vi "Rectifier Log Process.vi"   [LabVIEW 2019]
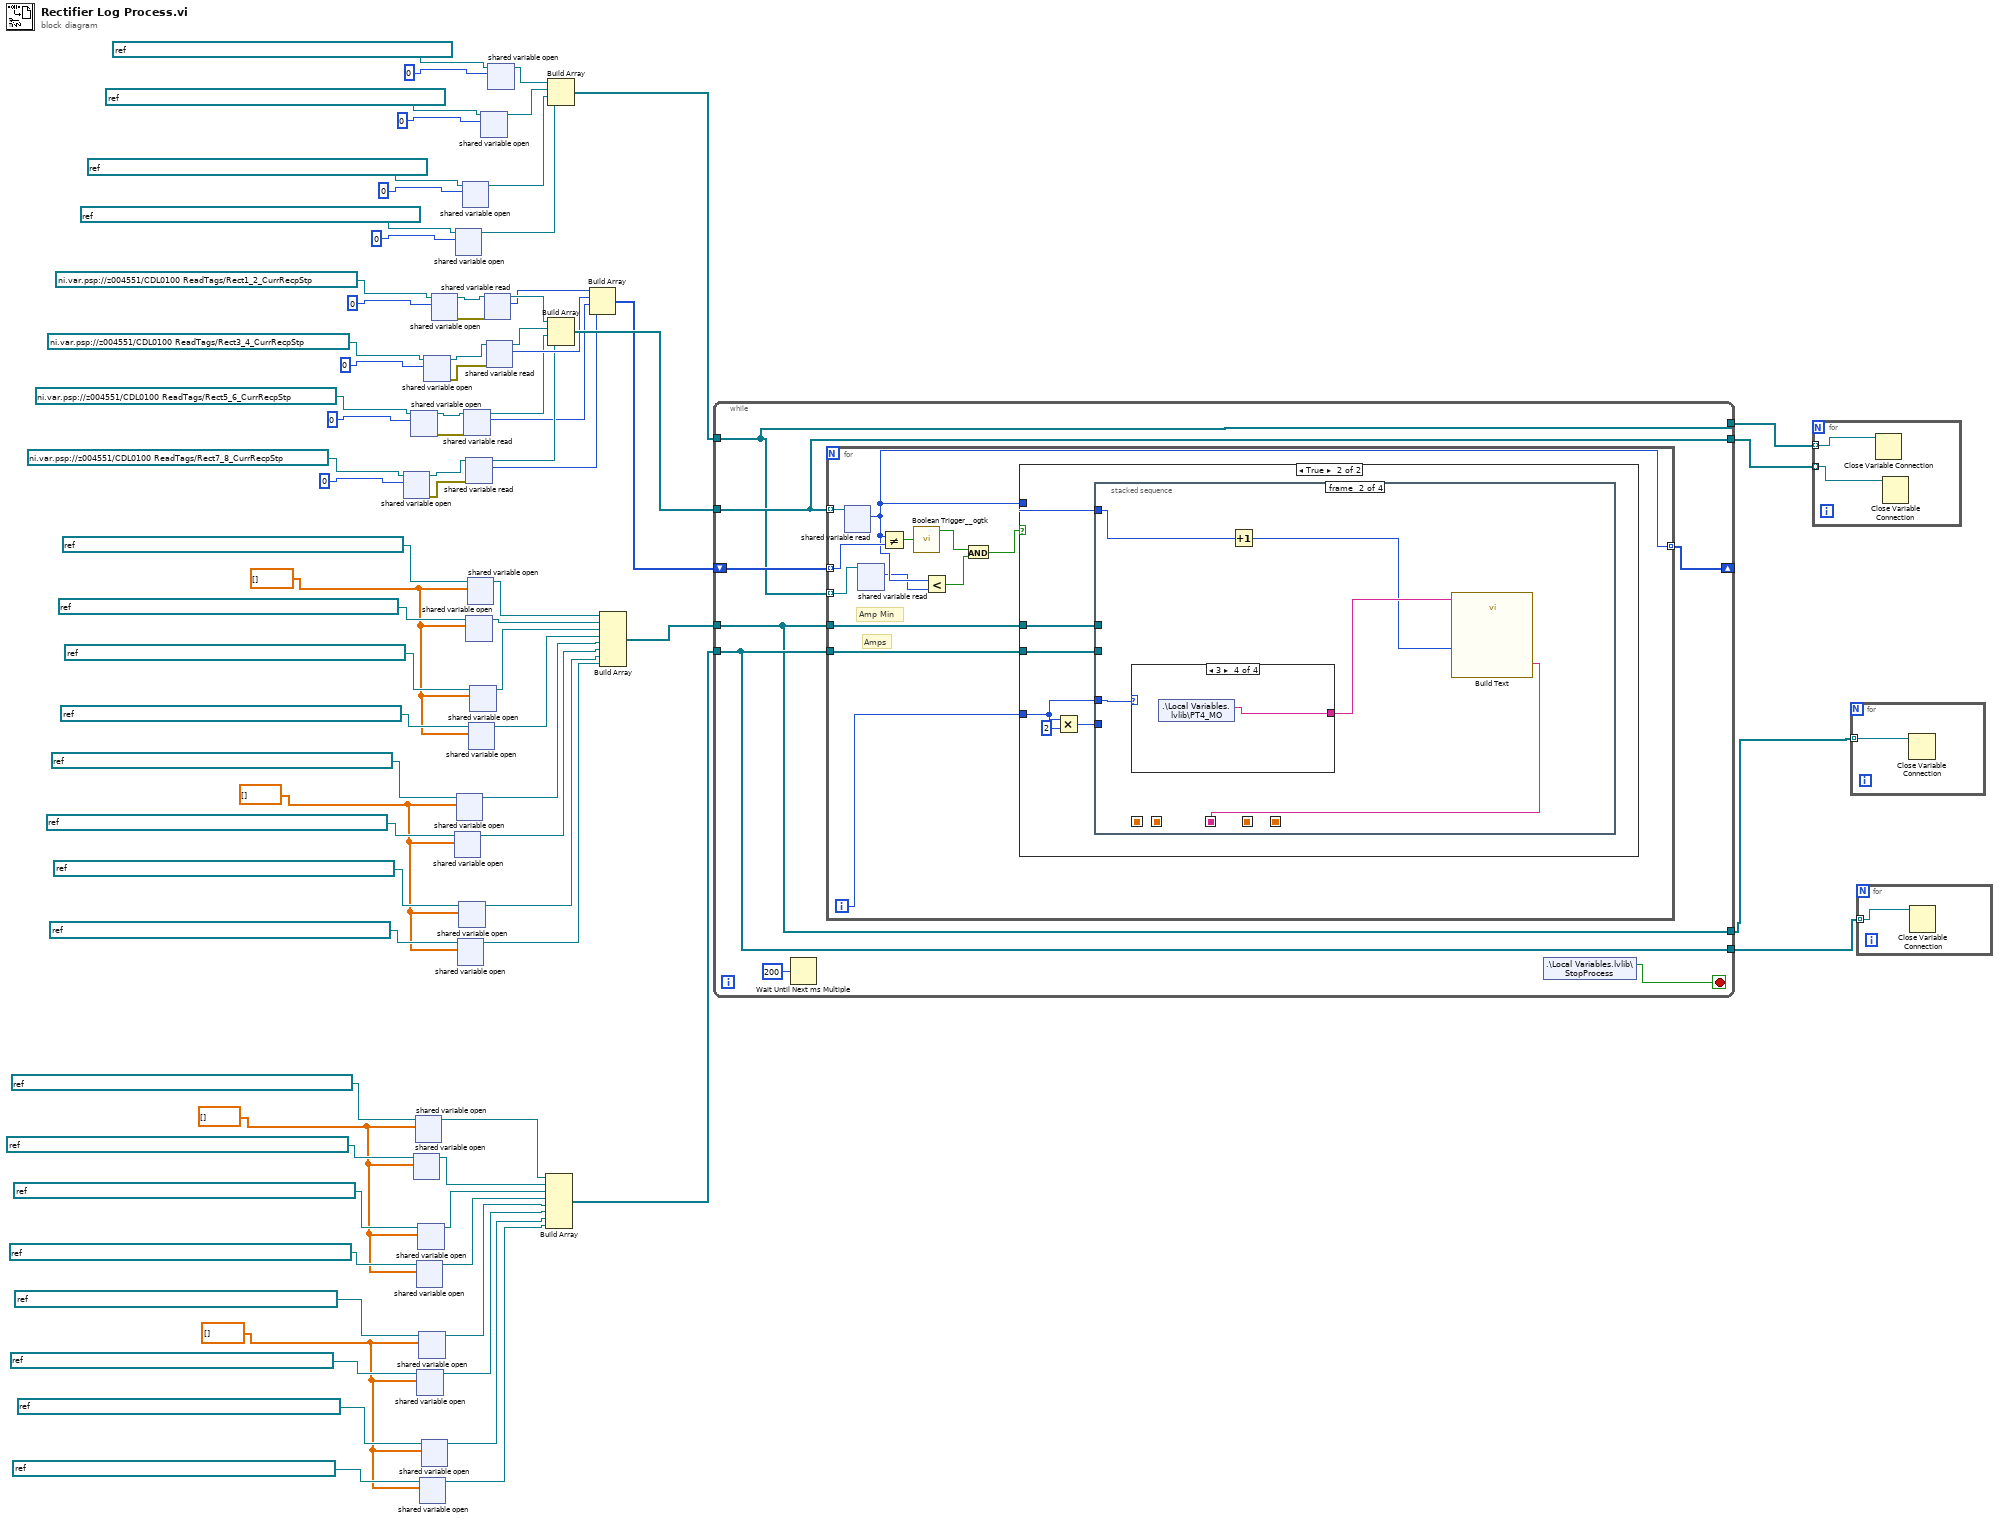
[diagram p0: block diagram]
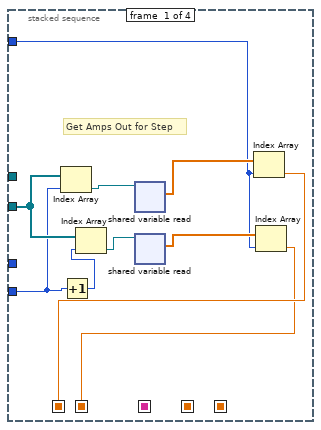
[diagram p3: hidden frame]
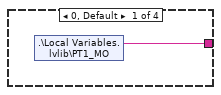
[diagram p4: hidden frame]
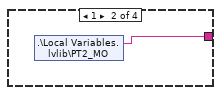
[diagram p5: hidden frame]
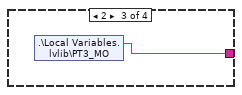
[diagram p6: hidden frame]
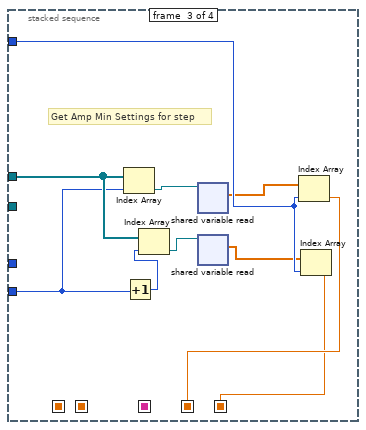
[diagram p7: hidden frame]
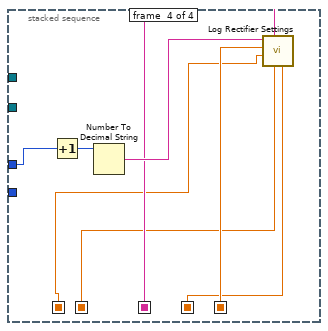
[diagram p8: hidden frame]
diagram:
  w5 = dbl[] []
  w14 = dbl[] []
  w64 = dbl[] []
  w73 = dbl[] []
  n1 = shared-variable-open(refnum<k21> "ni.var.psp://z004551/CDL0100 ReadTags/Rect7_8_CurrRecpStp" ("shared variable refnum in"), 0) -> (w24:refnum<k21>, w23:errorcluster)  [unwired: 2 in]
  n2 = shared-variable-open(refnum<k21> "ni.var.psp://z004551/CDL0100 ReadTags/Rect5_6_CurrRecpStp" ("shared variable refnum in"), 0) -> (w26:refnum<k21>, w25:errorcluster)  [unwired: 2 in]
  n3 = shared-variable-open(refnum<k21> "ni.var.psp://z004551/CDL0100 ReadWriteTags/HMI_Rct2_AFwd_SetPnts" ("shared variable refnum in"), w64) -> (w62:refnum<k21>)  [unwired: 2 in, 1 out]
  n4 = shared-variable-open(refnum<k21> "ni.var.psp://z004551/CDL0100 ReadWriteTags/HMI_Rct1_AFwd_SetPnts" ("shared variable refnum in"), w64) -> (w63:refnum<k21>)  [unwired: 2 in, 1 out]
  n5 = shared-variable-open(refnum<k21> "ni.var.psp://z004551/CDL0100 ReadWriteTags/HMI_Rct4_AFwd_SetPnts" ("shared variable refnum in"), w64) -> (w60:refnum<k21>)  [unwired: 2 in, 1 out]
  n6 = shared-variable-open(refnum<k21> "ni.var.psp://z004551/CDL0100 ReadWriteTags/HMI_Rct6_A_SetPnts" ("shared variable refnum in"), w5) -> (w3:refnum<k21>)  [unwired: 2 in, 1 out]
  n7 = shared-variable-open(refnum<k21> "ni.var.psp://z004551/CDL0100 ReadWriteTags/HMI_Rct3_AFwd_SetPnts" ("shared variable refnum in"), w64) -> (w61:refnum<k21>)  [unwired: 2 in, 1 out]
  n8 = shared-variable-open(refnum<k21> "ni.var.psp://z004551/CDL0100 ReadWriteTags/HMI_Rct5_A_SetPnts" ("shared variable refnum in"), w5) -> (w4:refnum<k21>)  [unwired: 2 in, 1 out]
  n9 = shared-variable-open(refnum<k21> "ni.var.psp://z004551/CDL0100 ReadWriteTags/HMI_Rct8_A_SetPnts" ("shared variable refnum in"), w5) -> (w1:refnum<k21>)  [unwired: 2 in, 1 out]
  n10 = shared-variable-open(refnum<k21> "ni.var.psp://z004551/CDL0100 ReadWriteTags/HMI_Rct7_A_SetPnts" ("shared variable refnum in"), w5) -> (w2:refnum<k21>)  [unwired: 2 in, 1 out]
  n11 = shared-variable-open(refnum<k21> "ni.var.psp://z004551/CDL0100 ReadTags/Rect3_4_CurrRecpStp" ("shared variable refnum in"), 0) -> (w54:refnum<k21>, w53:errorcluster)  [unwired: 2 in]
  n12 = shared-variable-open(refnum<k21> "ni.var.psp://z004551/CDL0100 ReadTags/Rect1_2_CurrRecpStp" ("shared variable refnum in"), 0) -> (w58:refnum<k21>, w56:errorcluster)  [unwired: 2 in]
  n13 = shared-variable-open(refnum<k21> "ni.var.psp://z004551/CDL0100 ReadWriteTags/HMI_Rct6_AMin_SetPnts" ("shared variable refnum in"), w14) -> (w12:refnum<k21>)  [unwired: 2 in, 1 out]
  n14 = shared-variable-open(refnum<k21> "ni.var.psp://z004551/CDL0100 ReadWriteTags/HMI_Rect7_8_NumSteps" ("shared variable refnum in"), 0) -> (w31:refnum<k21>)  [unwired: 2 in, 1 out]
  n15 = shared-variable-open(refnum<k21> "ni.var.psp://z004551/CDL0100 ReadWriteTags/HMI_Rct5_AMin_SetPnts" ("shared variable refnum in"), w14) -> (w13:refnum<k21>)  [unwired: 2 in, 1 out]
  n16 = shared-variable-open(refnum<k21> "ni.var.psp://z004551/CDL0100 ReadWriteTags/HMI_Rct8_AMin_SetPnts" ("shared variable refnum in"), w14) -> (w10:refnum<k21>)  [unwired: 2 in, 1 out]
  n17 = shared-variable-open(refnum<k21> "ni.var.psp://z004551/CDL0100 ReadWriteTags/HMI_Rct7_AMin_SetPnts" ("shared variable refnum in"), w14) -> (w11:refnum<k21>)  [unwired: 2 in, 1 out]
  n18 = shared-variable-open(refnum<k21> "ni.var.psp://z004551/CDL0100 ReadWriteTags/HMI_Rect5_6_NumSteps" ("shared variable refnum in"), 0) -> (w32:refnum<k21>)  [unwired: 2 in, 1 out]
  n19 = shared-variable-read(w26, w25) -> (w22:refnum<k21>, w20:i32)  [unwired: 2 out]
  n20 = shared-variable-read(w24, w23) -> (w21:refnum<k21>, w19:i32)  [unwired: 2 out]
  n21 = shared-variable-open(refnum<k21> "ni.var.psp://z004551/CDL0100 ReadWriteTags/HMI_Rct2_AMin_SetPnts" ("shared variable refnum in"), w73) -> (w71:refnum<k21>)  [unwired: 2 in, 1 out]
  n22 = shared-variable-open(refnum<k21> "ni.var.psp://z004551/CDL0100 ReadWriteTags/HMI_Rct1_AMin_SetPnts" ("shared variable refnum in"), w73) -> (w72:refnum<k21>)  [unwired: 2 in, 1 out]
  n23 = shared-variable-open(refnum<k21> "ni.var.psp://z004551/CDL0100 ReadWriteTags/HMI_Rct4_AMin_SetPnts" ("shared variable refnum in"), w73) -> (w69:refnum<k21>)  [unwired: 2 in, 1 out]
  n24 = shared-variable-open(refnum<k21> "ni.var.psp://z004551/CDL0100 ReadWriteTags/HMI_Rct3_AMin_SetPnts" ("shared variable refnum in"), w73) -> (w70:refnum<k21>)  [unwired: 2 in, 1 out]
  n25 = shared-variable-open(refnum<k21> "ni.var.psp://z004551/CDL0100 ReadWriteTags/HMI_Rect3_4_NumSteps" ("shared variable refnum in"), 0) -> (w39:refnum<k21>)  [unwired: 2 in, 1 out]
  n26 = shared-variable-read(w58, w56) -> (w57:refnum<k21>, w55:i32)  [unwired: 2 out]
  n27 = shared-variable-read(w54, w53) -> (w52:refnum<k21>, w51:i32)  [unwired: 2 out]
  n28 = shared-variable-open(refnum<k21> "ni.var.psp://z004551/CDL0100 ReadWriteTags/HMI_Rect1_2_NumSteps" ("shared variable refnum in"), 0) -> (w40:refnum<k21>)  [unwired: 2 in, 1 out]
  n29 = Build Array(w63, w62, w61, w60, w4, w3, w2, w1) -> (w48:refnum<k21>[])
  n30 = Build Array(w40, w39, w32, w31) -> (w38:refnum<k21>[])
  n31 = Build Array(w57, w52, w22, w21) -> (w59:refnum<k21>[])
  n32 = Build Array(w55, w51, w20, w19) -> (w50:i32[])
  n33 = Build Array(w72, w71, w70, w69, w13, w12, w11, w10) -> (w49:refnum<k21>[])
  n34 = while {
    tunnel: w59 -> [w85]
    shift-right: [w86] -> _
    shift-left: w50 -> [w87]
    tunnel: w49 -> [w83]
    tunnel: w48 -> [w84]
    tunnel: [w85] -> w47
    tunnel: [w84] -> w45
    tunnel: [w83] -> w46
    tunnel: w38 -> [w82]
    tunnel: [w82] -> w37
    stop <- w89 stop-if-true
    n35 = Wait Until Next ms Multiple(millisecond multiple=u32 200) -> ()  [unwired: 1 out]
    n36 = for {
      tunnel: w85 -> [w101] mode=indexing
      tunnel: w87 -> [w100] mode=indexing
      tunnel: [w94] -> w86 mode=indexing
      tunnel: w83 -> [w98]
      tunnel: w84 -> [w96]
      tunnel: w82 -> [w95] mode=indexing
      i -> [w97]
      # "Amps"
      # "Amp Min"
      n37 = shared-variable-read(w101) -> (w94:i32)  [unwired: 1 in, 3 out]
      n38 = shared-variable-read(w95) -> (w93:i32)  [unwired: 1 in, 3 out]
      n39 = Not Equal?(x=w94, y=w100) -> (x != y?=w99:bool)
      n40 = call <userlib>:"Boolean Trigger__ogtk.vi"("Boolean Input"=w99) -> ("Rising Edge"=w92:bool)  [unwired: 1 in, 1 out]
      n41 = Less?(x=w94, y=w93) -> (x < y?=w91:bool)
      n42 = And(x=w92, y=w91) -> (x .and. y?=w90:bool)
      n43 = case shown="True" w90 {
        tunnel: w98 -> [_ w102]
        tunnel: w96 -> [_ w105]
        tunnel: w94 -> [_ w104]
        tunnel: w97 -> [_ w103]
        frame False {
        }
        frame True {
          n44 = Multiply(x=w103, y=2) -> (x*y=w106:i32)
          n45 = stacked-sequence {
            seq-local: [w109 _ _ _] -> [_ _ _ w139]
            seq-local: [w108 _ _ _] -> [_ _ _ w138]
            seq-local: [_ w118 _ _] -> [_ _ _ w141]
            seq-local: [_ _ w128 _] -> [_ _ _ w137]
            seq-local: [_ _ w127 _] -> [_ _ _ w140]
            tunnel: w105 -> [w117 _ _ _]
            tunnel: w106 -> [w115 _ w132 _]
            tunnel: w104 -> [w110 w120 w131 _]
            tunnel: w103 -> [_ w122 _ w144]
            tunnel: w102 -> [_ _ w133 _]
            frame #0 {
              # "Get Amps Out for Step"
              n46 = Index Array(array=w117, index=w115) -> (element=w114:refnum<k21>)
              n47 = Increment(x=w115) -> (x+1=w116:i32)
              n48 = Index Array(array=w117, index=w116) -> (element=w113:refnum<k21>)
              n49 = shared-variable-read(w114) -> (w112:dbl[])  [unwired: 1 in, 3 out]
              n50 = shared-variable-read(w113) -> (w111:dbl[])  [unwired: 1 in, 3 out]
              n51 = Index Array(array=w112, index=w110) -> (element=w109:dbl)
              n52 = Index Array(array=w111, index=w110) -> (element=w108:dbl)
            }
            frame #1 {
              n53 = case shown="3" w122 {
                tunnel: [w123 w124 w125 w126] -> w121
                frame 0, Default {
                  n54 = shared-variable ".\\Local Variables.lvlib\\PT1_MO"() -> (w123:string)  [unwired: 1 in, 1 out]
                }
                frame 1 {
                  n55 = shared-variable ".\\Local Variables.lvlib\\PT2_MO"() -> (w124:string)  [unwired: 1 in, 1 out]
                }
                frame 2 {
                  n56 = shared-variable ".\\Local Variables.lvlib\\PT3_MO"() -> (w125:string)  [unwired: 1 in, 1 out]
                }
                frame 3 {
                  n57 = shared-variable ".\\Local Variables.lvlib\\PT4_MO"() -> (w126:string)  [unwired: 1 in, 1 out]
                }
              }
              n58 = Increment(x=w120) -> (x+1=w119:i32)
              n59 = call "Build Text"("Beginning Text"=w121, "d"=w119) -> ("Result"=w118:string)  [unwired: 12 in, 1 out]
            }
            frame #2 {
              # "Get Amp Min Settings for step"
              n60 = Index Array(array=w133, index=w132) -> (element=w135:refnum<k21>)
              n61 = Increment(x=w132) -> (x+1=w136:i32)
              n62 = Index Array(array=w133, index=w136) -> (element=w134:refnum<k21>)
              n63 = shared-variable-read(w135) -> (w130:dbl[])  [unwired: 1 in, 3 out]
              n64 = shared-variable-read(w134) -> (w129:dbl[])  [unwired: 1 in, 3 out]
              n65 = Index Array(array=w130, index=w131) -> (element=w128:dbl)
              n66 = Index Array(array=w129, index=w131) -> (element=w127:dbl)
            }
            frame #3 {
              n67 = Increment(x=w144) -> (x+1=w143:i32)
              n68 = Number To Decimal String(number=w143) -> (decimal integer string=w142:string)  [unwired: 1 in]
              n69 = call "Log Rectifier Settings.vi"("Amp-min Left Anode"=w137, "Right Anode Output"=w138, "Panel Name"=w141, "Left Anode Output"=w139, "Amp-min Right Anode"=w140, "Tank Number"=w142) -> ()  [unwired: 5 in, 1 out]
            }
          }
        }
      }
    }
    n70 = shared-variable ".\\Local Variables.lvlib\\StopProcess"() -> (w89:bool)  [unwired: 1 in, 1 out]
  }
  n71 = for {
    tunnel: w47 -> [w146] mode=indexing
    tunnel: w37 -> [w145] mode=indexing
    n72 = Close Variable Connection(11:w145) -> ()  [unwired: 1 in, 1 out]
    n73 = Close Variable Connection(11:w146) -> ()  [unwired: 1 in, 1 out]
  }
  n74 = for {
    tunnel: w46 -> [w147] mode=indexing
    n75 = Close Variable Connection(11:w147) -> ()  [unwired: 1 in, 1 out]
  }
  n76 = for {
    tunnel: w45 -> [w148] mode=indexing
    n77 = Close Variable Connection(11:w148) -> ()  [unwired: 1 in, 1 out]
  }
